vi "Ctor.vi"(8 "error in (no error)":errorcluster, 11 "Class In":refnum<class "Rate Step.lvclass">) -> (0 "error out":errorcluster, 3 "Class":refnum<class "Rate Step.lvclass">)   [LabVIEW 2018, in "Temp Recipe.lvlib" / "Rate Step.lvclass"]
uses:
  Rate Step.lvclass
  Ref Data.ctl
  Rate Step.lvclass/Rate Step.ctl
  Recipe Step/Recipe Step.lvclass
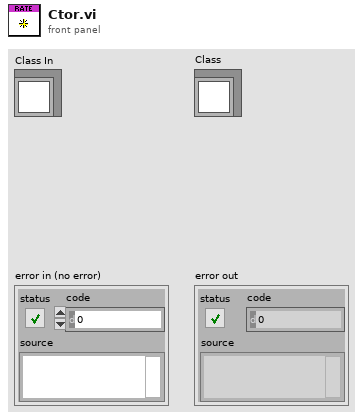
[diagram p1: front panel]
types:
  T1 = typedef "Temp Recipe.lvlib/Rate Step.lvclass/Ref Data.ctl" = cluster{"Step Temp":dbl, "Step Time":dbl, "Target":dbl}
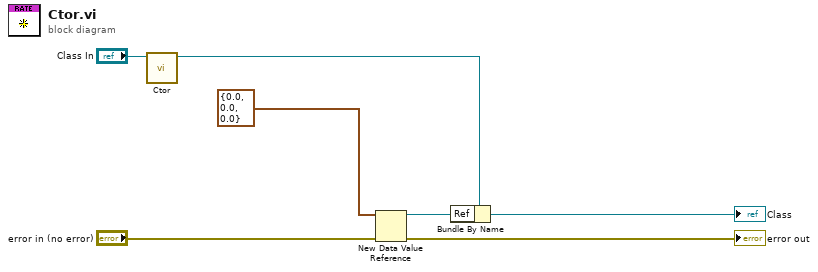
[diagram p0: block diagram]
diagram:
  n1 = call-parent "Ctor.vi"("Panel in"="Class In") -> ("Panel out"=w1:refnum<class "Rate Step.lvclass">)  [unwired: 9 in, 1 out]
  n2 = New Data Value Reference(data value=T1 {"Step Temp"=0.0, "Step Time"=0.0, "Target"=0.0} ("Ref Data"), error in="error in (no error)") -> (data value reference=w4:refnum<data-value>, error out=→"error out":errorcluster)
  n3 = Bundle By Name(cluster=w1, "Ref"=w4) -> (→"Class":refnum<class "Rate Step.lvclass">)
